vi "start.vi"(8 "error in (no error)":errorcluster, 11 "TemperatureSensor in":refnum<class "TemperatureSensor.lvclass">) -> (0 "error out":errorcluster, 3 "TemperatureSensor out":refnum<class "TemperatureSensor.lvclass">)   [LabVIEW 2013, in "TemperatureSensor.lvclass"]
uses:
  TemperatureSensor.lvclass
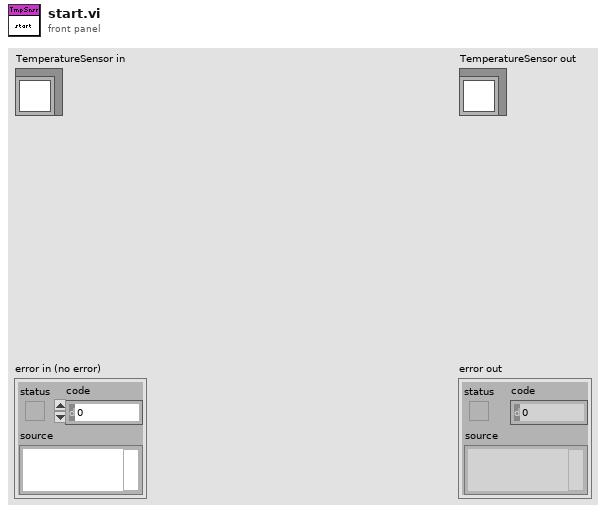
[diagram p1: front panel]
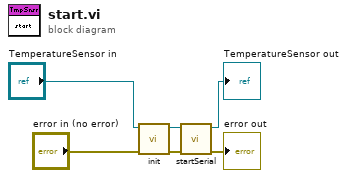
[diagram p0: block diagram]
diagram:
  n1 = call-dynamic "init.vi"("error in (no error)"="error in (no error)", "TemperatureSensor in"="TemperatureSensor in") -> ("error out"=w2:errorcluster, "TemperatureSensor out"=w3:refnum<class "TemperatureSensor.lvclass">)  [unwired: 8 in]
  n2 = call "startSerial.vi"("error in (no error)"=w2, "TemperatureSensor in"=w3) -> ("error out"=→"error out":errorcluster, "TemperatureSensor out"=→"TemperatureSensor out":refnum<class "TemperatureSensor.lvclass">)  [unwired: 8 in]
